vi "Protocol Read to CRLF.vi"(8 "error in":errorcluster, 9 "timeout":i32=10000, 10 "bytes to read":i32, 11 "protocol layer in":refnum<class "Serial Slave.lvclass">) -> (0 "error out":errorcluster, 1 "timed out?":bool, 2 "data":u8[](array[numeric]), 3 "protocol layer out":refnum<class "Serial Slave.lvclass">)   [LabVIEW 2021]
doc: "This provides an interface for reading from a network bus."
uses:
  Serial Slave.lvclass
  Serial Slave.lvclass/Serial Slave.ctl
  Serial Shared Components/Serial Shared Components.lvlib
  D:/my_projects/projects/Algorithms/Labview/21/Modbus_v121c/Network Protocol/Network Slave/Network Slave.lvclass
  D:/my_projects/projects/Algorithms/Labview/21/Modbus_v121c/Network Protocol/Network Protocol.lvclass
  D:/my_projects/projects/Algorithms/Labview/21/Modbus_v121c/Network Protocol/Network Slave/Serial/Serial Slave.lvclass
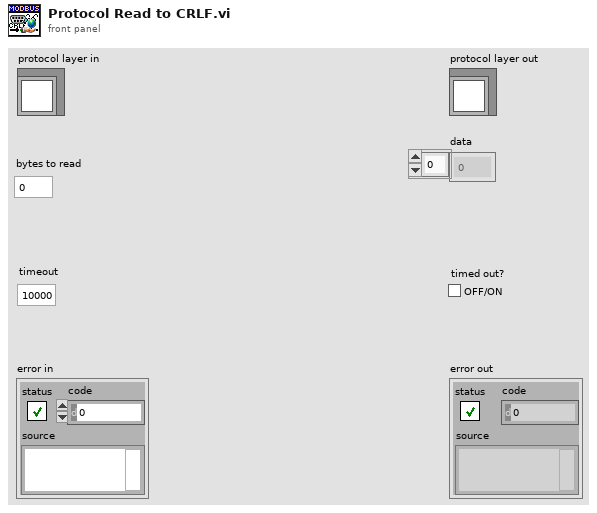
[diagram p1: front panel]
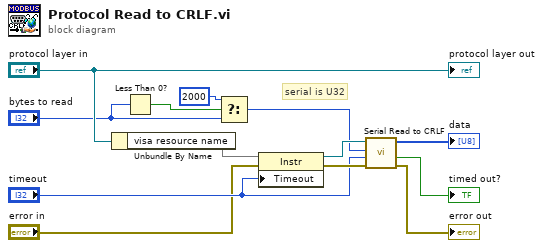
[diagram p0: block diagram]
diagram:
  # "serial is U32"
  n1 = Unbundle By Name("protocol layer in") -> ("visa resource name"=w11)
  n2 = Less Than 0?(x="bytes to read") -> (x < 0?=w13:bool)
  n3 = Select(t=u32 2000, s=w13, f="bytes to read") -> (s? t:f=w8:u32)
  n4 = property class="Instr"(reference=w11, error in="error in", "Timeout"="timeout") -> (reference out=w9:refnum<visa-resource-name>, error out=w10:errorcluster)
  n5 = call "Serial Read to CRLF.vi"("error in"=w10, "timeout (ms)"="timeout", "bytes to read"=w8, "Visa Resource"=w9) -> ("error out"=→"error out":errorcluster, "timed out?"=→"timed out?":bool, "data"=→"data":u8[])  [unwired: 5 in]
  "protocol layer out" <- "protocol layer in"
